vi "Attenuator_Close.vi"(3 "error in (no error)":errorcluster caption="错误输入（无错误）") -> (0 "error out":errorcluster caption="错误输出")   [LabVIEW 2018]
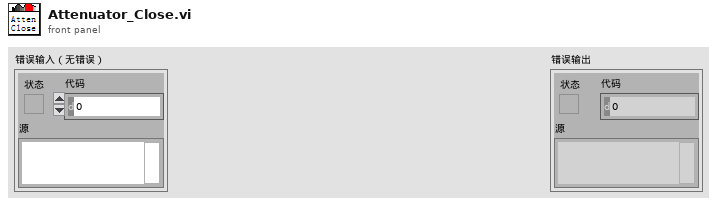
[diagram p1: front panel]
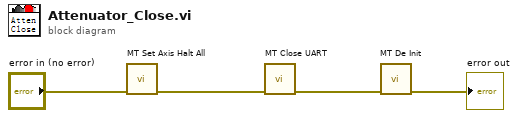
[diagram p0: block diagram]
diagram:
  n1 = call "MT Set Axis Halt All.vi"("error in (no error)"="error in (no error)") -> ("error out"=w2:errorcluster)  [unwired: 9 in, 1 out]
  n2 = call "MT Close UART.vi"("error in (no error)"=w2) -> ("error out"=w1:errorcluster)  [unwired: 9 in, 1 out]
  n3 = call "MT De Init.vi"("error in (no error)"=w1) -> ("error out"=→"error out":errorcluster)  [unwired: 9 in, 1 out]
